vi "Setup UI.vi"(8 "error in (no error)":errorcluster, 11 "Operator UI in":refnum<class "Measurement Setup UI.lvclass">) -> (0 "error out":errorcluster, 3 "Operator UI out":refnum<class "Measurement Setup UI.lvclass">)   [LabVIEW 2015, in "Measurement Setup Controller.lvlib" / "Measurement Setup UI.lvclass"]
uses:
  Measurement Setup UI.lvclass
  Measurement Setup UI.lvclass/Measurement Setup UI.ctl
  <userlib>/Common Components/Msmt UI/Measurement UI.lvclass/Measurement UI.ctl
  Read Save.vi
  <userlib>/Common Components/Msmt UI/Accessors/Read Run.vi
  <userlib>/Common Components/Msmt UI/Measurement UI.lvclass
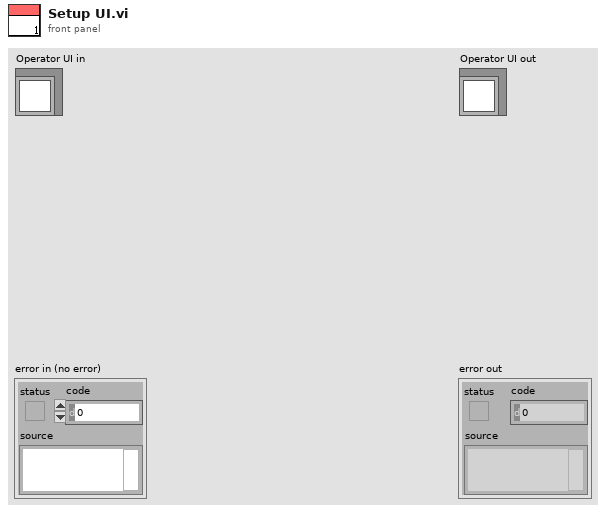
[diagram p1: front panel]
types:
  T1 = enum8{"Enabled", "Disabled", "Disabled and Grayed Out"}
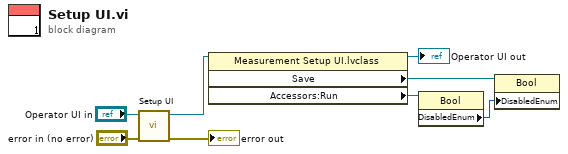
[diagram p0: block diagram]
diagram:
  n1 = call-parent "Setup UI.vi"("error in (no error)"="error in (no error)", "Operator UI in"="Operator UI in") -> ("error out"=→"error out":errorcluster, "Operator UI out"=w8:refnum<class "Measurement Setup UI.lvclass">)  [unwired: 8 in]
  n2 = property class="Measurement Setup UI.lvclass"(reference=w8) -> (reference out=→"Operator UI out":refnum<class "Measurement Setup UI.lvclass">, "Save"=w3:refnum<vi>, "Accessors:Run"=w2:refnum<vi>)  [unwired: 1 in, 1 out]
  n3 = property class="Bool"(reference=w2) -> ("DisabledEnum"=w4:T1)  [unwired: 1 in, 2 out]
  n4 = property class="Bool"(reference=w3, "DisabledEnum"=w4) -> ()  [unwired: 1 in, 2 out]
